vi "Receive Labels.vi"() -> ()   [LabVIEW 2019]
doc: "This program opens the specified card, configures the first receive channel from the configuration file with filters set for 2 messages and a default filter. Then the message data is continuously read and displayed."
uses:
  <instrlib>/BTICardLib/Private/Initialize By Card Number and Core Number.vi
  <instrlib>/BTICardLib/Private/Configure Core From XML.vi
  <instrlib>/BTI429Lib/Private/Rx/Configure/Configure Rx Channel From XML.vi
  <instrlib>/BTI429Lib/Private/Rx/Configure/Get Rx Label Handle Name.vi
  <instrlib>/BTI429Lib/Private/Core/Action-Status/Start Channel.vi
  <instrlib>/BTI429Lib/Private/Core/Action-Status/Stop Channel.vi
  <instrlib>/BTICardLib/BTICardLV.lvlib
  <instrlib>/BTI429Lib/BTI429LV.lvlib
panel:
  out "rx channel number":i32
  out "core number":i32
  out "error out":errorcluster
  in  "Channel Configuration XML file name":string="Channel Config.xml"
  in  "Core Configuration XML file name":string="Core Config.xml"
  in  "Card Number":i32
  out "Data 2":u32 format="%x"
  out "Data 1":u32 format="%x"
  out "Default":u32 format="%x"
  in  "stop":bool
  # "ARINC 429: Receive Labels"
  # "©2016 Astronics Ballard Technology"
  # "This program opens the specified card, configures the first receive channel from the configuration file with filters set for 2 messages and a default filter. Then the message data is continuously read and displayed."
  # "This labels for Data 1 and Data 2\nare defined in the Channel XML\nConfiguration. Shipping defaults\nare Label 206 and 211."
  # "Always Stop the card\nand Close the card when\ndone. Otherwise, the hardware\ncontinues to operate."
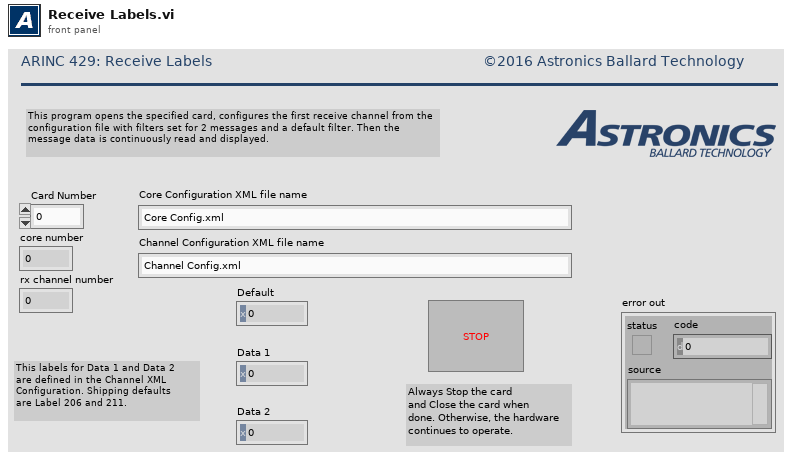
[diagram p1: front panel]
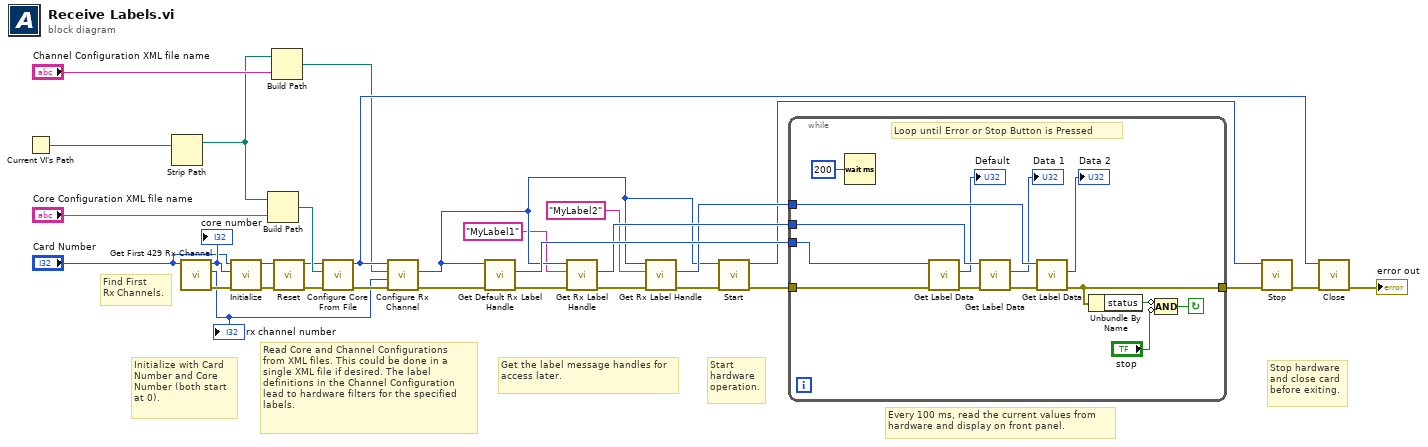
[diagram p0: block diagram]
diagram:
  # "Find First  \nRx Channels."
  # "Stop hardware\nand close card\nbefore exiting."
  # "Every 100 ms, read the current values from \nhardware and display on front panel."
  # "Start\nhardware\noperation."
  # "Get the label message handles for access later."
  # "Read Core and Channel Configurations\nfrom XML files. This could be done in a\nsingle XML file if desired. The label \ndefinitions in the Channel Configuration\nlead to hardware filters for the specified\nlabels."
  # "Initialize with Card\nNumber and Core\nNumber (both start\nat 0)."
  n1 = Current VI's Path() -> (path=w14:path)
  n2 = Strip Path(path=w14) -> (stripped path=w11:path)  [unwired: 1 out]
  n3 = call "Get First 429 Rx Channel.vi"("Card Number"="Card Number") -> ("error out"=w4:errorcluster, "Channel Number"=w1:i32, "Core Number"=w3:i32)  [unwired: 8 in]
  "core number" <- w3
  "rx channel number" <- w1
  n4 = call-poly <instrlib>:"Initialize.vi"("error in (no error)"=w4, "core number"=w3, "card number"="Card Number") -> ("error out"=w5:errorcluster, "core handle out"=w8:u64)  [unwired: 7 in]
  n5 = Build Path(base path=w11, name or relative path="Core Configuration XML file name") -> (appended path=w9:path)
  n6 = Build Path(base path=w11, name or relative path="Channel Configuration XML file name") -> (appended path=w12:path)
  n7 = call <instrlib>:"Reset.vi"("error in (no error)"=w5, "core handle in"=w8) -> ("error out"=w6:errorcluster, "core handle out"=w7:u64)  [unwired: 8 in]
  n8 = call-poly <instrlib>:"Configure Core From File.vi"("error in (no error)"=w6, "configuration file path"=w9, "core handle in"=w7) -> ("error out"=w20:errorcluster, "core handle out"=w16:u64)  [unwired: 7 in]
  n9 = call-poly <instrlib>:"Configure Rx Channel.vi"("error in (no error)"=w20, "channel number in"=w1, "configuration file path"=w12, "core handle in"=w16) -> ("error out"=w31:errorcluster, "channel handle out"=w23:u64)  [unwired: 5 in, 1 out]
  n10 = call <instrlib>:"Get Default Rx Label Handle.vi"("error in (no error)"=w31, "channel handle in"=w23) -> ("error out"=w30:errorcluster, "default label handle out"=w26:u64)  [unwired: 7 in, 1 out]
  n11 = call-poly <instrlib>:"Get Rx Label Handle.vi"("error in (no error)"=w30, "label name"="MyLabel1", "channel handle in"=w23) -> ("error out"=w29:errorcluster, "label handle out"=w25:u64)  [unwired: 6 in, 1 out]
  n12 = call-poly <instrlib>:"Get Rx Label Handle.vi"("error in (no error)"=w29, "label name"="MyLabel2", "channel handle in"=w23) -> ("error out"=w28:errorcluster, "label handle out"=w24:u64)  [unwired: 6 in, 1 out]
  n13 = call-poly <instrlib>:"Start.vi"("error in (no error)"=w28, "channel handle in"=w23) -> ("error out"=w27:errorcluster, "channel handle out"=w21:u64)  [unwired: 8 in]
  n14 = while {
    tunnel: w27 -> [w33]
    tunnel: w26 -> [w41]
    tunnel: w25 -> [w40]
    tunnel: w24 -> [w39]
    tunnel: [w34] -> w15
    stop <- w45 continue-if-true
    # "Loop until Error or Stop Button is Pressed"
    n15 = Wait (ms)(milliseconds to wait=u32 200) -> ()  [unwired: 1 out]
    n16 = call <instrlib>:"Get Label Data.vi"("error in (no error)"=w33, "label handle in"=w41) -> ("error out"=w42:errorcluster, "value"=→"Default":u32)  [unwired: 7 in, 1 out]
    n17 = call <instrlib>:"Get Label Data.vi"("error in (no error)"=w42, "label handle in"=w40) -> ("error out"=w43:errorcluster, "value"=→"Data 1":u32)  [unwired: 7 in, 1 out]
    n18 = call <instrlib>:"Get Label Data.vi"("error in (no error)"=w43, "label handle in"=w39) -> ("error out"=w34:errorcluster, "value"=→"Data 2":u32)  [unwired: 7 in, 1 out]
    n19 = Unbundle By Name(w34) -> ("status"=w35:bool)
    n20 = Compound Arithmetic op=AND(invert w35, invert "stop") -> (w45:bool)
  }
  n21 = call-poly <instrlib>:"Stop.vi"("error in (no error)"=w15, "channel handle in"=w21) -> ("error out"=w22:errorcluster)  [unwired: 8 in, 1 out]
  n22 = call <instrlib>:"Close.vi"("error in (no error)"=w22, "core handle in"=w16) -> ("error out"=→"error out":errorcluster)  [unwired: 8 in, 1 out]
